vi "Configure Front Panel Layouts.vi"(8 "error in":errorcluster, 9 "VIs to exclude":string[](array[string]), 10 "close window when done? (F)":bool) -> (0 "error out":errorcluster)   [LabVIEW 2012, in "NI_SE_Config Front Panel Layout.lvlib"]
uses:
  NI_SE_Config Front Panel Layout.lvlib
panel:
  in  "include size":bool
  in  "keyword":string caption="Keyword"
  in  "help":bool
  in  "load":bool
  in  "save":bool
  in  "refresh":bool
  in  "remove VI":bool
  in  "add VI":bool
  in  "configs":string[](tree) caption="VI Configurations"
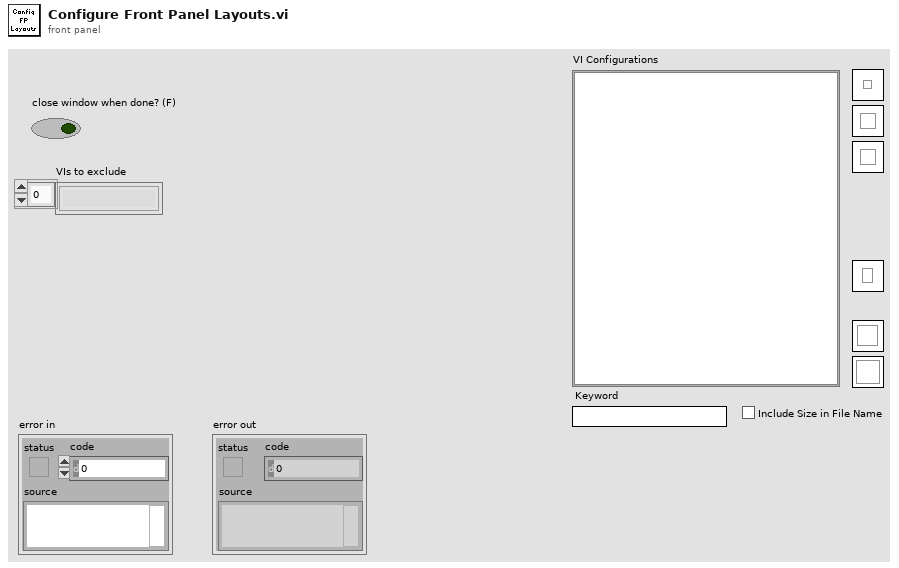
[diagram p1: front panel]
types:
  T1 = typedef "NI_SE_Config Front Panel Layout.lvlib/State.ctl" = cluster{"dialog VI refnum":refnum<vi>, "tree refnum":refnum<vi>, "VI info":T2[], "VI info list":variant, "subpanel tags":variant}
  T2 = typedef "NI_SE_Config Front Panel Layout.lvlib/VI Info.ctl" = cluster{"VI ref":refnum<vi>, "panel layout":refnum<class "VI Panel Layout.lvclass">, "tree tag":string, "parent tag":string, "subpanel refs":variant}
  T3 = cluster{"data name":string, "drag data":variant}[]
  T4 = typedef "LVPoint32TypeDef.ctl" = cluster{"Horizontal":i32, "Vertical":i32}
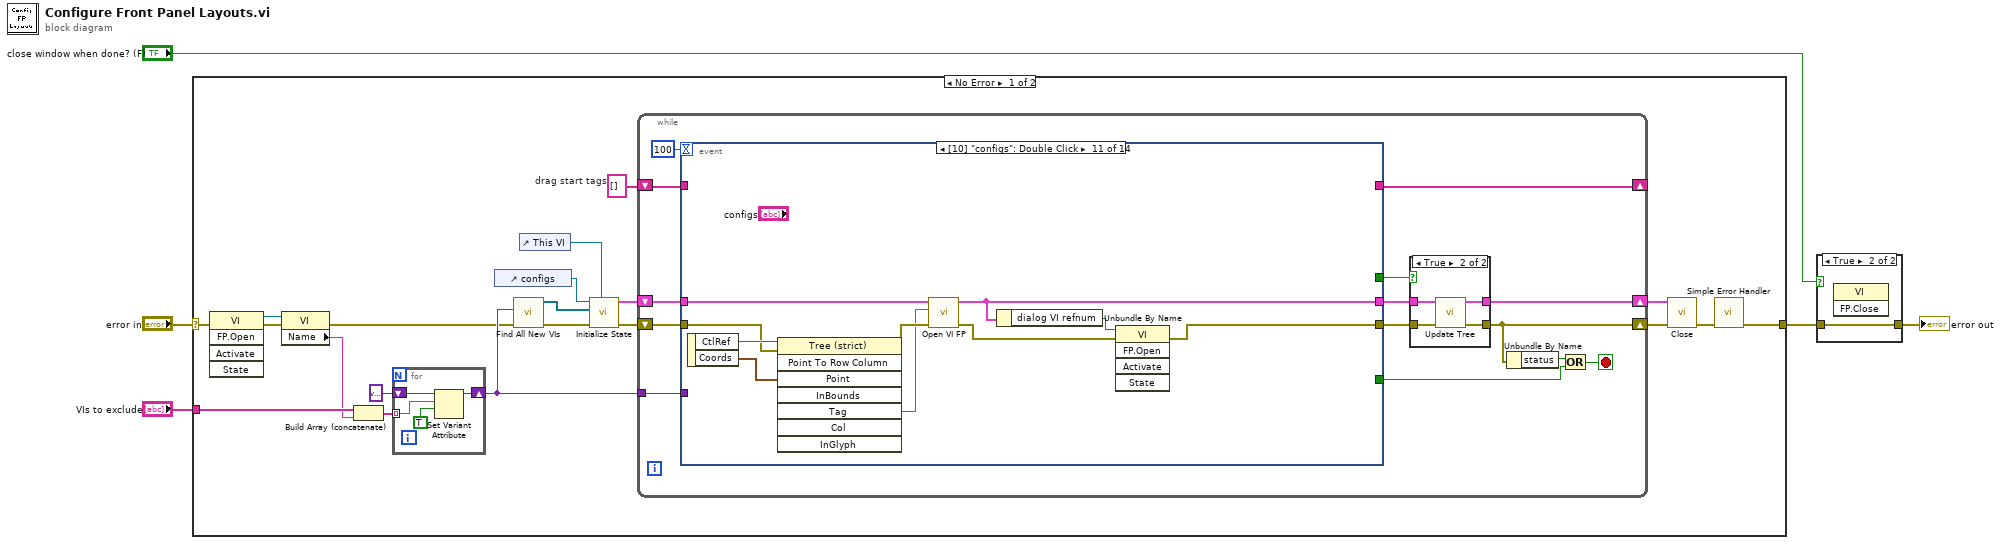
[diagram p0: block diagram]
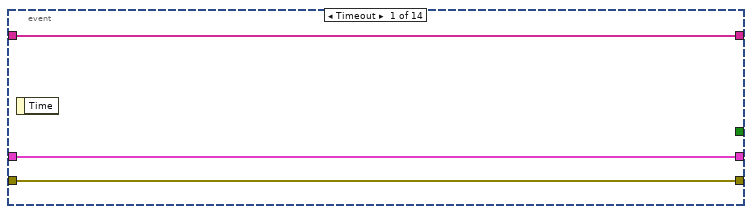
[diagram p4: hidden frame]
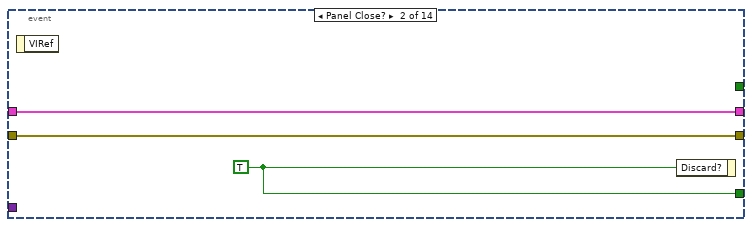
[diagram p5: hidden frame]
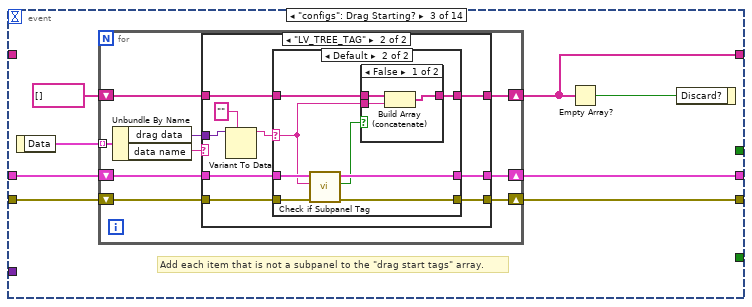
[diagram p6: hidden frame]
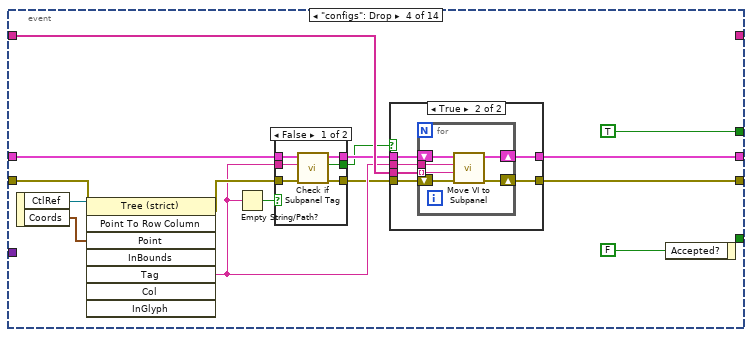
[diagram p10: hidden frame]
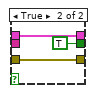
[diagram p11: hidden frame]
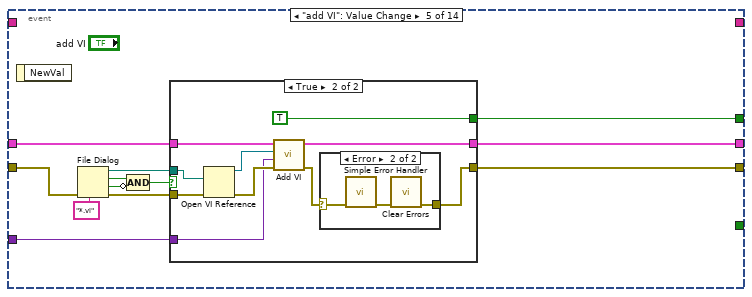
[diagram p13: hidden frame]
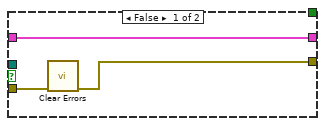
[diagram p14: hidden frame]
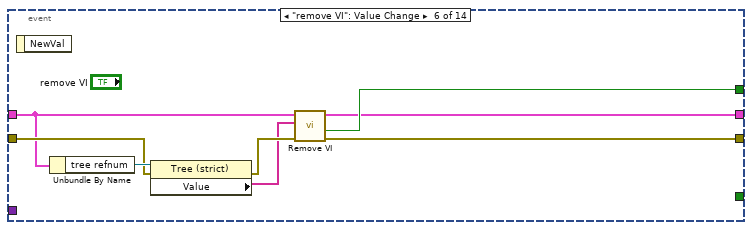
[diagram p16: hidden frame]
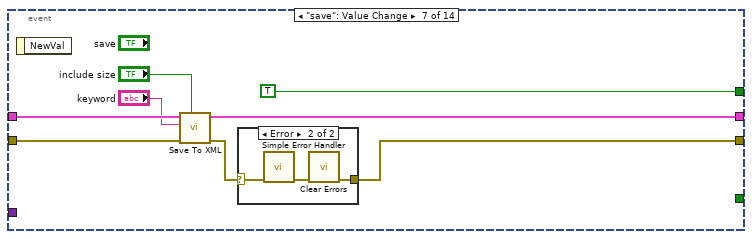
[diagram p17: hidden frame]
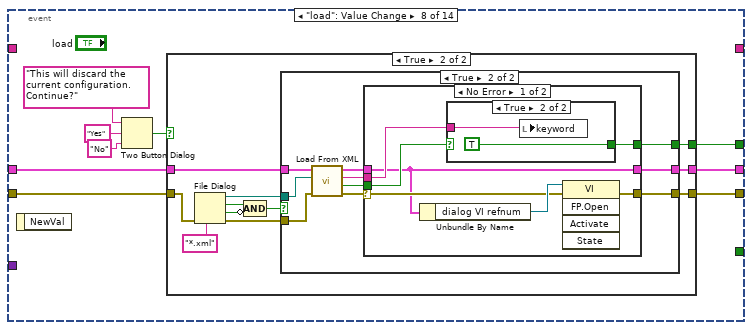
[diagram p19: hidden frame]
diagram:
  n1 = case shown="No Error" "error in" {
    selector: "error in" -> [w11 w286]
    tunnel: [w20 w286] -> w4
    tunnel: "VIs to exclude" -> [w18 _]
    frame No Error {
      w12 = string[] []  # drag start tags
      n2 = invoke class="VI" method="FP.Open"(error in=w11) -> (reference out=w19:refnum<vi>, error out=w10:errorcluster)  [unwired: 4 in, 3 out]
      n3 = property class="VI"(reference=w19, error in=w10) -> (error out=w6:errorcluster, "Name"=w17:string)  [unwired: 1 out]
      n4 = Build Array (concatenate)(w18, w17) -> (w16:string[])
      n5 = for {
        tunnel: w16 -> [w27] mode=indexing
        shift-right: [w29] -> w9
        shift-left: variant -> [w28]
        n6 = Set Variant Attribute(Variant=w28, name=w27, value=TRUE) -> (Variant out=w29:variant)  [unwired: 1 in, 2 out]
      }
      n7 = control-ref of="configs"() -> (w13:refnum<vi>)
      n8 = call "Find All New VIs.vi"("error in"=w6, "VIs  to exclude"=w9) -> ("error out"=w7:errorcluster, "VI refs"=w8:refnum<vi>[])  [unwired: 8 in]
      n9 = control-ref of="This VI"() -> (w14:refnum<vi>)
      n10 = call "Initialize State.vi"("dialog VI refnum"=w14, "error in"=w7, "VI refs"=w8, "tree refnum"=w13) -> ("error out"=w24:errorcluster, "state out"=w25:T1)  [unwired: 6 in]
      n11 = while {
        shift-right: [w33] -> w21
        shift-left: w25 -> [w40]
        shift-right: [w35] -> w23
        shift-left: w24 -> [w39]
        shift-right: [w38] -> _
        shift-left: w12 -> [w37]
        tunnel: w9 -> [w31]
        stop <- w41 stop-if-true
        n12 = event shown="[10] \"configs\": Double Click" {
          selector: _ -> [_ _ _ _ _ _ _ _ _ _ _ _ _ _]
          dyn-events: _ -> [_ _ _ _ _ _ _ _ _ _ _ _ _ _]
          timeout: 100 -> [_ _ _ _ _ _ _ _ _ _ _ _ _ _]
          tunnel: w39 -> [w52 w55 w61 w112 w145 w173 w180 w195 w238 w251 w262 w267 w274 w284]
          tunnel: [w52 w55 w59 w108 w147 w170 w175 w193 w243 w250 w255 w267 w269 w276] -> w36
          tunnel: [_ w54 _ _ _ _ _ _ _ _ _ _ _ _] -> w42
          tunnel: w40 -> [w51 w53 w62 w111 w149 w172 w182 w194 w244 w253 w261 w266 w275 w285]
          tunnel: [w51 w53 w60 w107 w148 w167 w181 w192 w244 w252 w257 w266 w270 w279] -> w34
          tunnel: [w50 _ w58 _ _ _ _ _ _ _ _ _ _ _] -> w38
          tunnel: w37 -> [w50 _ _ w109 _ _ _ _ _ _ _ _ _ _]
          tunnel: [_ _ _ TRUE w142 w169 TRUE w187 _ TRUE _ _ _ w280] -> w32
          tunnel: w31 -> [_ _ _ _ w138 _ _ _ _ w249 _ _ _ _]
          event Timeout {
            n13 = event-data() -> ()  [unwired: 1 in, 1 out]
          }
          event Panel Close? {
            w54 = TRUE ("Discard?")
            n14 = event-data() -> ()  [unwired: 1 in, 1 out]
            n15 = event-data("Discard?"=w54) -> ()  [unwired: 1 in, 1 out]
          }
          event "configs": Drag Starting? {
            # "Add each item that is not a subpanel to the \"drag start tags\" array."
            n16 = event-data() -> ("Data"=w63:T3)  [unwired: 1 in]
            n17 = for {
              tunnel: w63 -> [w72] mode=indexing
              shift-right: [w68] -> w60
              shift-left: w62 -> [w70]
              shift-right: [w67] -> w59
              shift-left: w61 -> [w69]
              shift-right: [w64] -> w58
              shift-left: string[] [] -> [w65]
              n18 = Unbundle By Name(w72) -> ("drag data"=w71:variant, "data name"=w66:string)
              n19 = case shown="\"LV_TREE_TAG\"" w66 {
                tunnel: w71 -> [_ w84]
                tunnel: w70 -> [w75 w82]
                tunnel: w69 -> [w74 w80]
                tunnel: [w75 w81] -> w68
                tunnel: [w74 w79] -> w67
                tunnel: w65 -> [w73 w78]
                tunnel: [w73 w77] -> w64
                frame Default {
                }
                frame "LV_TREE_TAG" {
                  n20 = Variant To Data(type="", Variant=w84) -> (data=w76:string)  [unwired: 1 in, 1 out]
                  n21 = case shown="Default" w76 {
                    selector: w76 -> [_ w88]
                    tunnel: w82 -> [w86 w95]
                    tunnel: [w86 w94] -> w81
                    tunnel: w80 -> [w85 w93]
                    tunnel: [w85 w92] -> w79
                    tunnel: w78 -> [w87 w90]
                    tunnel: [w87 w89] -> w77
                    frame "" {
                    }
                    frame Default {
                      n22 = call "Check if Subpanel Tag.vi"("error in"=w93, "subpanel tag"=w88, "state in"=w95) -> ("error out"=w92:errorcluster, "found?"=w91:bool, "state out"=w94:T1)  [unwired: 4 in, 2 out]
                      n23 = case shown="False" w91 {
                        tunnel: w88 -> [w97 _]
                        tunnel: w90 -> [w98 w99]
                        tunnel: [w96 w99] -> w89
                        frame False {
                          n24 = Build Array (concatenate)(w98, w97) -> (w96:string[])
                        }
                        frame True {
                        }
                      }
                    }
                  }
                }
              }
            }
            n25 = Empty Array?(array=w58) -> (empty?=w57:bool)
            n26 = event-data("Discard?"=w57) -> ()  [unwired: 1 in, 1 out]
          }
          event "configs": Drop {
            n27 = event-data() -> ("CtlRef"=w113:refnum<vi>, "Coords"=w114:T4)  [unwired: 1 in]
            n28 = invoke class="Tree (strict)" method="Point To Row Column"(reference=w113, error in=w112, "Point"=w114) -> (error out=w110:errorcluster, "Tag"=w104:string)  [unwired: 5 in, 6 out]
            n29 = Empty String/Path?(string/path=w104) -> (empty?=w100:bool)
            n30 = case shown="False" w100 {
              tunnel: w111 -> [w120 w123]
              tunnel: w110 -> [w119 w122]
              tunnel: w104 -> [w118 _]
              tunnel: [w117 w123] -> w103
              tunnel: [w116 w122] -> w102
              tunnel: [w115 TRUE ("found?")] -> w101
              frame False {
                n31 = call "Check if Subpanel Tag.vi"("error in"=w119, "subpanel tag"=w118, "state in"=w120) -> ("error out"=w116:errorcluster, "found?"=w115:bool, "state out"=w117:T1)  [unwired: 4 in, 2 out]
              }
              frame True {
              }
            }
            n32 = case shown="True" w101 {
              tunnel: w109 -> [_ w131]
              tunnel: w103 -> [w125 w130]
              tunnel: w102 -> [w124 w129]
              tunnel: [w124 w128] -> w108
              tunnel: [w125 w127] -> w107
              tunnel: w104 -> [_ w126]
              frame False {
              }
              frame True {
                n33 = for {
                  tunnel: w131 -> [w137] mode=indexing
                  tunnel: w126 -> [w132]
                  shift-right: [w134] -> w128
                  shift-left: w129 -> [w135]
                  shift-right: [w133] -> w127
                  shift-left: w130 -> [w136]
                  n34 = call "Move VI to Subpanel.vi"("error in"=w135, "VI name"=w137, "subpanel tag"=w132, "state in"=w136) -> ("error out"=w134:errorcluster, "state out"=w133:T1)  [unwired: 6 in]
                }
              }
            }
            n35 = event-data("Accepted?"=FALSE) -> ()  [unwired: 1 in, 1 out]
          }
          event "add VI": Value Change {
            n36 = event-data() -> ()  [unwired: 1 in, 1 out]
            n37 = File Dialog(6:"*.vi" ("pattern (all files)"), 8:w145) -> (0:w143:errorcluster, 1:w140:bool, 2:w141:bool, 3:w144:path)  [unwired: 5 in]
            n38 = Compound Arithmetic op=AND(w141, invert w140) -> (w139:bool)
            n39 = case shown="True" w139 {
              tunnel: w149 -> [w152 w156]
              tunnel: [w152 w162] -> w148
              tunnel: [w150 w153] -> w147
              tunnel: w144 -> [_ w161]
              tunnel: w143 -> [w151 w160]
              tunnel: [_ TRUE] -> w142
              tunnel: w138 -> [_ w155]
              frame False {
                n40 = call <vilib>:"Clear Errors.vi"("error in (no error)"=w151) -> ("error out"=w150:errorcluster)  [unwired: 6 in]
              }
              frame True {
                n41 = Open VI Reference(vi path=w161, error in (no error)=w160) -> (vi reference=w158:refnum<vi>, error out=w159:errorcluster)  [unwired: 4 in]
                n42 = call "Add VI.vi"("error in"=w159, "VIs to exclude"=w155, "VI ref"=w158, "state in"=w156) -> ("error out"=w154:errorcluster, "state out"=w162:T1)  [unwired: 6 in]
                n43 = case shown="Error" w154 {
                  selector: w154 -> [w163 w166]
                  tunnel: [w163 w164] -> w153
                  frame No Error {
                  }
                  frame Error {
                    n44 = call <vilib>:"Simple Error Handler.vi"("error in (no error)"=w166) -> ("error out"=w165:errorcluster)  [unwired: 4 in, 4 out]
                    n45 = call <vilib>:"Clear Errors.vi"("error in (no error)"=w165) -> ("error out"=w164:errorcluster)  [unwired: 6 in]
                  }
                }
              }
            }
          }
          event "remove VI": Value Change {
            n46 = event-data() -> ()  [unwired: 1 in, 1 out]
            n47 = Unbundle By Name(w172) -> ("tree refnum"=w174:refnum<vi>)
            n48 = property class="Tree (strict)"(reference=w174, error in=w173) -> (error out=w171:errorcluster, "Value"=w168:string[])  [unwired: 1 out]
            n49 = call "Remove VI.vi"("error in"=w171, "VI names"=w168, "state in"=w172) -> ("error out"=w170:errorcluster, "removed?"=w169:bool, "state out"=w167:T1)  [unwired: 6 in]
          }
          event "save": Value Change {
            n50 = event-data() -> ()  [unwired: 1 in, 1 out]
            n51 = call "Save To XML.vi"("include size in file name? (F)"="include size", "error in"=w180, "layout keyword"="keyword", "state in"=w182) -> ("error out"=w176:errorcluster, "state out"=w181:T1)  [unwired: 6 in]
            n52 = case shown="Error" w176 {
              selector: w176 -> [w183 w186]
              tunnel: [w183 w184] -> w175
              frame No Error {
              }
              frame Error {
                n53 = call <vilib>:"Simple Error Handler.vi"("error in (no error)"=w186) -> ("error out"=w185:errorcluster)  [unwired: 4 in, 4 out]
                n54 = call <vilib>:"Clear Errors.vi"("error in (no error)"=w185) -> ("error out"=w184:errorcluster)  [unwired: 6 in]
              }
            }
          }
          event "load": Value Change {
            n55 = event-data() -> ()  [unwired: 1 in, 1 out]
            n56 = Two Button Dialog(message="This will discard the current configuration.  Continue?", 1:"No" ("F button name (\"Cancel\")"), 2:"Yes" ("T button name (\"OK\")")) -> (T button?=w188:bool)
            n57 = case shown="True" w188 {
              tunnel: w195 -> [w196 w202]
              tunnel: w194 -> [w197 w201]
              tunnel: [w196 w200] -> w193
              tunnel: [w197 w199] -> w192
              tunnel: [_ w198] -> w187
              frame False {
              }
              frame True {
                n58 = File Dialog(6:"*.xml" ("pattern (all files)"), 8:w202) -> (0:w206:errorcluster, 1:w204:bool, 2:w205:bool, 3:w207:path)  [unwired: 5 in]
                n59 = Compound Arithmetic op=AND(w205, invert w204) -> (w203:bool)
                n60 = case shown="True" w203 {
                  tunnel: w201 -> [w211 w220]
                  tunnel: [w211 w212] -> w199
                  tunnel: [w209 w214] -> w200
                  tunnel: w207 -> [_ w216]
                  tunnel: w206 -> [w210 w219]
                  tunnel: [_ w221] -> w198
                  frame False {
                    n61 = call <vilib>:"Clear Errors.vi"("error in (no error)"=w210) -> ("error out"=w209:errorcluster)  [unwired: 6 in]
                  }
                  frame True {
                    n62 = call "Load From XML.vi"("error in"=w219, "XML file path"=w216, "state in"=w220) -> ("error out"=w213:errorcluster, "loaded?"=w218:bool, "layout keyword"=w217:string, "state out"=w215:T1)  [unwired: 5 in]
                    n63 = case shown="No Error" w213 {
                      selector: w213 -> [w223 w234]
                      tunnel: [w228 TRUE] -> w221
                      tunnel: w218 -> [w227 _]
                      tunnel: w217 -> [w226 _]
                      tunnel: w215 -> [w222 w235]
                      tunnel: [w225 w232] -> w214
                      tunnel: [w222 w235] -> w212
                      frame No Error {
                        n64 = Unbundle By Name(w222) -> ("dialog VI refnum"=w224:refnum<vi>)
                        n65 = case shown="True" w227 {
                          tunnel: [_ TRUE] -> w228
                          tunnel: w226 -> [_ w229]
                          frame False {
                          }
                          frame True {
                            n66 = local write "keyword"(w229) -> ()
                          }
                        }
                        n67 = invoke class="VI" method="FP.Open"(reference=w224, error in=w223) -> (error out=w225:errorcluster)  [unwired: 3 in, 4 out]
                      }
                      frame Error {
                        n68 = call <vilib>:"Simple Error Handler.vi"("error in (no error)"=w234) -> ("error out"=w233:errorcluster)  [unwired: 4 in, 4 out]
                        n69 = call <vilib>:"Clear Errors.vi"("error in (no error)"=w233) -> ("error out"=w232:errorcluster)  [unwired: 6 in]
                      }
                    }
                  }
                }
              }
            }
          }
          event "help": Value Change {
            n70 = event-data() -> ()  [unwired: 1 in, 1 out]
            n71 = property class="App"() -> ("App.Dir"=w241:path)  [unwired: 2 in, 2 out]
            n72 = Build Path(base path=w241, name or relative path=path "manuals/Getting_Started_NI_FrontPanelLayout.pdf" ("Application:Directory Path")) -> (appended path=w240:path)
            n73 = call <vilib>:"Check if File or Folder Exists.vi"("error in (no error)"=w238, "path"=w240) -> ("error out"=w237:errorcluster, "file or folder exists?"=w236:bool, "dup path"=w239:path)  [unwired: 7 in]
            n74 = case shown="True" w236 {
              tunnel: [w245 w248] -> w243
              tunnel: w239 -> [_ w247]
              tunnel: w237 -> [w245 w246]
              frame False {
              }
              frame True {
                n75 = call <vilib>:"Open Acrobat Document.vi"("error in (no error)"=w246, "acrobat document"=w247) -> ("error out"=w248:errorcluster)  [unwired: 5 in]
              }
            }
          }
          event "refresh": Value Change {
            n76 = event-data() -> ()  [unwired: 1 in, 1 out]
            n77 = call "Refresh To Find New VIs.vi"("error in"=w251, "VIs  to exclude"=w249, "state in"=w253) -> ("error out"=w250:errorcluster, "state out"=w252:T1)  [unwired: 7 in]
          }
          event "configs": Double Click {
            n78 = event-data() -> ("CtlRef"=w263:refnum<vi>, "Coords"=w264:T4)  [unwired: 1 in]
            n79 = invoke class="Tree (strict)" method="Point To Row Column"(reference=w263, error in=w262, "Point"=w264) -> (error out=w260:errorcluster, "Tag"=w259:string)  [unwired: 5 in, 6 out]
            n80 = call "Open VI FP.vi"("error in"=w260, "VI name"=w259, "state in"=w261) -> ("error out"=w256:errorcluster, "state out"=w257:T1)  [unwired: 7 in]
            n81 = Unbundle By Name(w257) -> ("dialog VI refnum"=w258:refnum<vi>)
            n82 = invoke class="VI" method="FP.Open"(reference=w258, error in=w256) -> (error out=w255:errorcluster)  [unwired: 3 in, 4 out]
          }
          event "configs": event type 3.0.x80000011 {
            n83 = event-data() -> ()  [unwired: 1 in, 1 out]
            n84 = event-data("Discard?"=FALSE) -> ()  [unwired: 1 in, 1 out]
          }
          event "configs": Shortcut Menu Activation? {
            n85 = event-data() -> ("MenuRef"=w273:refnum<k9>, "CtlRef"=w272:refnum<vi>, "Coords"=w271:T4)  [unwired: 1 in]
            n86 = call "Handle Tree Shortcut Activation Event.vi"("Coords"=w271, "error in"=w274, "tree refnum"=w272, "menu reference"=w273, "state in"=w275) -> ("error out"=w269:errorcluster, "discard?"=w268:bool, "state out"=w270:T1)  [unwired: 4 in]
            n87 = event-data("Discard?"=w268) -> ()  [unwired: 1 in, 1 out]
          }
          event "configs": Shortcut Menu Selection (User) {
            n88 = event-data() -> ("ItemTag"=w283:string, "CtlRef"=w282:refnum<vi>, "Coords"=w281:T4)  [unwired: 1 in]
            n89 = call "Handle Tree Shortcut Selection Event.vi"("coords"=w281, "error in"=w284, "tree refnum"=w282, "ItemTag"=w283, "state in"=w285) -> ("error out"=w277:errorcluster, "update tree?"=w280:bool, "state out"=w279:T1)  [unwired: 4 in]
            n90 = Unbundle By Name(w279) -> ("dialog VI refnum"=w278:refnum<vi>)
            n91 = invoke class="VI" method="FP.Open"(reference=w278, error in=w277) -> (error out=w276:errorcluster)  [unwired: 3 in, 4 out]
          }
        }
        n92 = case shown="True" w32 {
          tunnel: w36 -> [w44 w48]
          tunnel: [w44 w46] -> w35
          tunnel: w34 -> [w45 w49]
          tunnel: [w45 w47] -> w33
          frame False {
          }
          frame True {
            n93 = call "Update Tree.vi"("error in"=w48, "state in"=w49) -> ("error out"=w46:errorcluster, "state out"=w47:T1)  [unwired: 8 in]
          }
        }
        n94 = Unbundle By Name(w35) -> ("status"=w30:bool)
        n95 = Or(x=w30, y=w42) -> (x .or. y?=w41:bool)
      }
      n96 = call "Close.vi"("error in"=w23, "state in"=w21) -> ("error out"=w22:errorcluster)  [unwired: 9 in]
      n97 = call <vilib>:"Simple Error Handler.vi"("error in (no error)"=w22) -> ("error out"=w20:errorcluster)  [unwired: 4 in, 4 out]
    }
    frame Error {
    }
  }
  n98 = case shown="True" "close window when done? (F)" {
    tunnel: w4 -> [w287 w288]
    tunnel: [w287 w288] -> w2
    frame False {
    }
    frame True {
      n99 = invoke class="VI" method="FP.Close"() -> ()  [unwired: 3 in, 3 out]
    }
  }
  "error out" <- w2
